vi "Express VI - Collector.vi"() -> ()   [LabVIEW 2023]
doc: "This example shows how to use the Collector Express VI. The Collector Express VI collects and returns input signals. You can specify the maximum number of samples the Collector can hold. When you call this Express VI repeatedly, as the While Loop in this example does, and the Express VI reaches the maximum number of samples per channel, the Express VI discards the oldest data and adds the newest data to the collected samples. This example shows the differences in collected data when you change the maximum number of samples."
panel:
  out "Number of Samples":i32
  in  "Send":bool
  in  "Stop":bool
  out "Collected Signal":dynamicdata(graph)
  out "Input Signal":dynamicdata(graph)
  # "Overview: Demonstrates the use of the Collector Express VI.\nInstructions:\n1. Run the VI.\n2. Click the Send button to send the Input Signal (10 samples) to the Collector.\n3. Click the Send button two more times and notice the Number of Samples in the Collected Signal does not increase above 25 because the Collector is configured to collect up to 25 samples.\n4. Click the Stop button to stop the VI.\n5. Open the block diagram. Right-click on the Collector Express VI and select Properties.\n6. Change the Maximum Number of Samples to 5.\n7. Run the VI again. Notice the Number of Samples in the Collected Signal does not increase above 5."
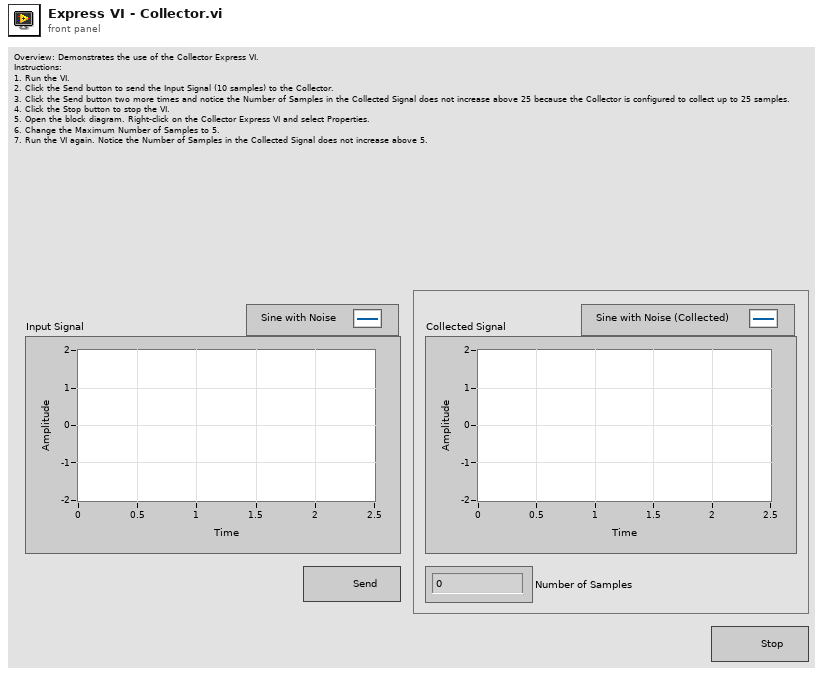
[diagram p1: front panel]
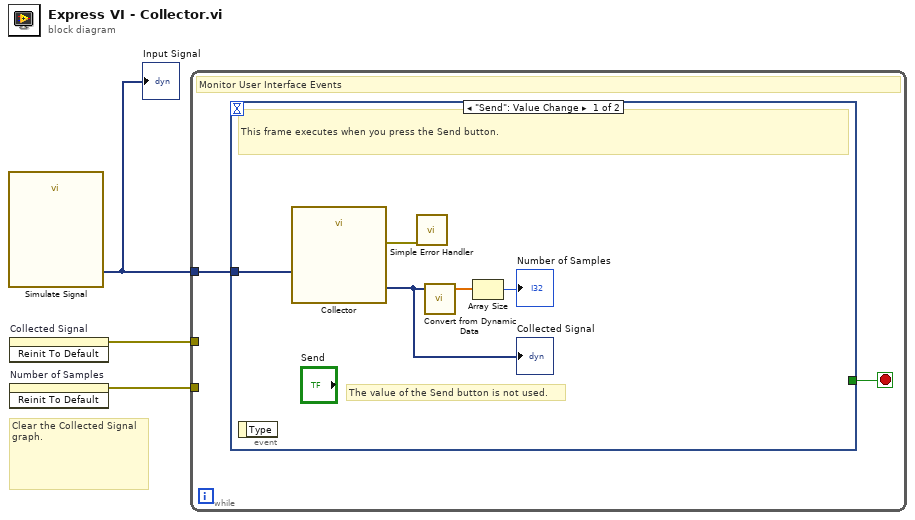
[diagram p0: block diagram]
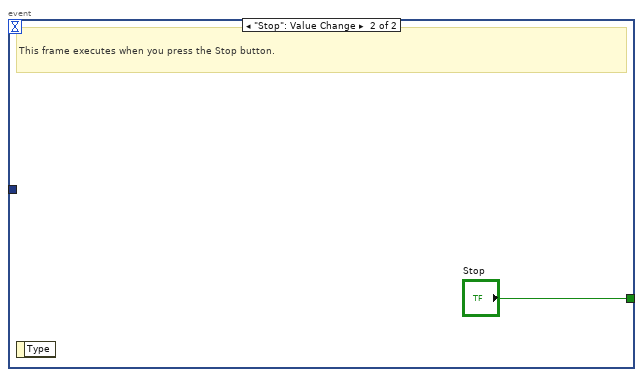
[diagram p2: hidden frame]
diagram:
  # "Clear the Collected Signal graph."
  n1 = call "Simulate Signal"() -> ("Sine with Noise"=w3:dynamicdata)  [unwired: 14 in, 1 out]
  "Input Signal" <- w3
  n2 = invoke on="Collected Signal" class="WFGraph (strict)" method="Reinit To Default"() -> (error out=w2:errorcluster)  [unwired: 3 in, 2 out]
  n3 = invoke on="Number of Samples" class="DigNum (strict)" method="Reinit To Default"() -> (error out=w1:errorcluster)  [unwired: 3 in, 2 out]
  n4 = while {
    tunnel: w3 -> [w4]
    tunnel: w2 -> [_]
    tunnel: w1 -> [_]
    stop <- w5 stop-if-true
    # "Monitor User Interface Events"
    n5 = event shown="[0] \"Send\": Value Change" {
      selector: _ -> [_ _]
      dyn-events: _ -> [_ _]
      timeout: _ -> [_ _]
      tunnel: [_ "Stop"] -> w5
      tunnel: w4 -> [w7 _]
      event "Send": Value Change {
        # "The value of the Send button is not used."
        # "This frame executes when you press the Send button."
        n6 = event-data() -> ()  [unwired: 1 in, 1 out]
        n7 = call "Collector"("Signals"=w7) -> ("error out"=w6:errorcluster, "Collected Signals"=w10:dynamicdata)  [unwired: 9 in]
        "Collected Signal" <- w10
        n8 = call <vilib>:"Simple Error Handler.vi"("error in (no error)"=w6) -> ()  [unwired: 4 in, 5 out]
        n9 = call "Convert from Dynamic Data"("Dynamic Data Type"=w10) -> ("Array"=w9:dbl[])  [unwired: 3 in]
        n10 = Array Size(array=w9) -> (size(s)=→"Number of Samples":i32)
      }
      event "Stop": Value Change {
        # "This frame executes when you press the Stop button."
        n11 = event-data() -> ()  [unwired: 1 in, 1 out]
      }
    }
  }
